vi "SmartMotor_Read EncRes an d Sampling Rate.vi"(8 "error in (no error)":errorcluster, 9 "ReadWait":u32=50, 10 "MotorSpecifier(M1)":T1, 11 "VISA Refnum in":refnum<visa-resource-name>) -> (0 "error out":errorcluster, 2 "SamplingRate":dbl, 3 "EncResolution":dbl)   [LabVIEW 2017]
doc: "Developed by Kevin Thompson\nkevin@thompsonengineering.net\n\nCopyright 2018-2020\nThompson Engineering, LLC"
uses:
  TD SerialBusMotorSpecifier_enum.ctl
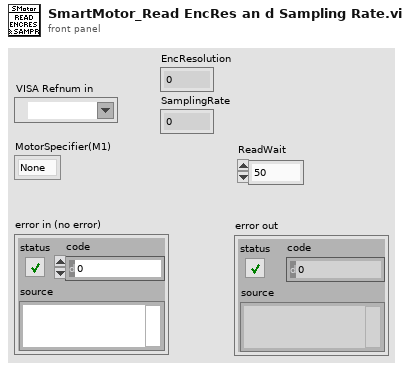
[diagram p1: front panel]
types:
  T1 = typedef "TD SerialBusMotorSpecifier_enum.ctl" = enum16{"None", "Global", "M1", "M2", "M3"}
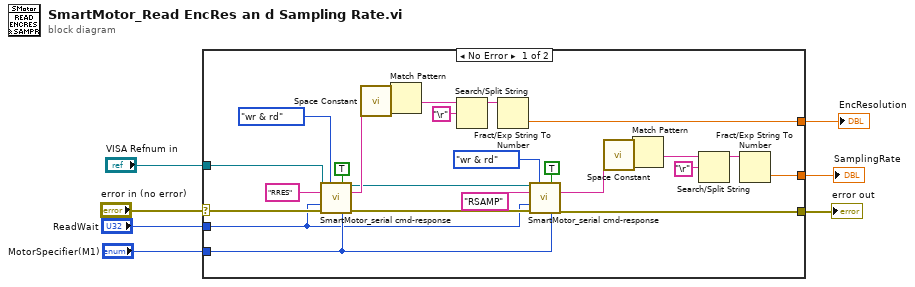
[diagram p0: block diagram]
diagram:
  n1 = case shown="No Error" "error in (no error)" {
    selector: "error in (no error)" -> [w9 w33]
    tunnel: "MotorSpecifier(M1)" -> [w22 _]
    tunnel: "VISA Refnum in" -> [w19 _]
    tunnel: [w13 _] -> w5
    tunnel: [w12 _] -> w4
    tunnel: [w10 w33] -> w3
    tunnel: "ReadWait" -> [w8 _]
    frame No Error {
      n2 = call "SmartMotor_serial cmd-response.vi"("VISA In"=w19, "mode"=enum16{"wr & rd", "write", "read"}."wr & rd", "flush transcvr(F)"=TRUE, "cmd"="RRES", "ReadWait"=w8, "error in"=w9, "MotorSpecifier(None)"=w22) -> ("VISA out"=w16:refnum<visa-resource-name>, "str out"=w24:string, "error out"=w11:errorcluster)  [unwired: 4 in, 2 out]
      n3 = call <vilib>:"Space Constant.vi"() -> ("String"=w23:string)
      n4 = Match Pattern(string=w24, regular expression=w23) -> (after substring=w25:string)  [unwired: 1 in, 3 out]
      n5 = Search/Split String(string=w25, search string/char (-)="\r") -> (substring before match=w15:string)  [unwired: 1 in, 2 out]
      n6 = Fract/Exp String To Number(string=w15) -> (number=w13:dbl)  [unwired: 3 in, 1 out]
      n7 = call "SmartMotor_serial cmd-response.vi"("VISA In"=w16, "mode"=enum16{"wr & rd", "write", "read"}."wr & rd", "flush transcvr(F)"=TRUE, "cmd"="RSAMP", "ReadWait"=w8, "error in"=w11, "MotorSpecifier(None)"=w22) -> ("str out"=w30:string, "error out"=w10:errorcluster)  [unwired: 4 in, 3 out]
      n8 = call <vilib>:"Space Constant.vi"() -> ("String"=w27:string)
      n9 = Match Pattern(string=w30, regular expression=w27) -> (after substring=w28:string)  [unwired: 1 in, 3 out]
      n10 = Search/Split String(string=w28, search string/char (-)="\r") -> (substring before match=w29:string)  [unwired: 1 in, 2 out]
      n11 = Fract/Exp String To Number(string=w29) -> (number=w12:dbl)  [unwired: 3 in, 1 out]
    }
    frame Error {
    }
  }
  "EncResolution" <- w5
  "SamplingRate" <- w4
  "error out" <- w3
